vi "ComputeClassicalCrossTalk.vi"() -> ()   [LabVIEW 2015]
uses:
  <vilib>/Utility/file.llb/Write Delimited Spreadsheet (DBL).vi
panel:
  in  "stop":bool
  out "SLM  B":picture
  out "SLM A":picture
  out "Cross Talk":dbl[][](array[numeric])=[[1.04866638e-09, 2.36400149e-10, 3.28397032e-10, 3.4456285e-11, 1.42615789e-11, 6.36260558e-11, 1.65061454e-11, 1.20186092e-11, 3.22117194e-11, 4.34313557e-11, 1.69085523e-10, -3.68856204e-12, 5.28650778e-12, -1.44559289e-12, 7.52947704e-12, 3.04194213e-12, 9.77404269e-12, 3.04194213e-12, 7.52947704e-12, 7.98972867e-13, 3.04194213e-12], [1.0401547e-10, 2.07185158e-09, 5.01172714e-10, 4.89953078e-10, 3.66992547e-11, 9.77404269e-12, 4.34313557e-11, 5.46509886e-11, 9.77404269e-12, 6.81135912e-11, 1.51135382e-10, 6.81135912e-11, 9.05512679e-11, 1.87491134e-11, 1.0625844e-10, 2.77241841e-11, 1.20186092e-11, 4.1188386e-11, 5.28650778e-12, 1.20186092e-11, 3.04194213e-12], [3.57566809e-10, 2.61082406e-10, 4.32914238e-09, 1.01725206e-09, 9.49937462e-10, 1.2645314e-10, 1.65061454e-11, 7.93332275e-11, 8.38207628e-11, 5.68939583e-11, 5.01634567e-11, 9.77404269e-12, 4.1188386e-11, 1.42615789e-11, 2.77241841e-11, 1.65061454e-11, 9.77404269e-12, 1.20186092e-11, 7.52947704e-12, 1.65061454e-11, 9.77404269e-12], [5.28650778e-12, 7.52481022e-10, 3.50836304e-10, 9.81754322e-09, 2.47574095e-09, 1.2820246e-09, 2.880092e-10, 7.03581568e-11, 5.46509886e-11, 1.1523351e-10, 7.26011265e-11, 1.65061454e-11, 1.87491134e-11, 1.87491134e-11, 6.81135912e-11, 1.42615789e-11, 1.87491134e-11, 7.52947704e-12, 5.28650778e-12, 7.52947704e-12, 1.87491134e-11], [2.32366487e-11, 3.89438204e-11, 1.28651212e-09, 5.43805057e-10, 2.64532805e-08, 3.65150532e-09, 1.94619743e-09, 2.16205456e-10, 3.35129119e-10, 7.26011265e-11, 1.51135382e-10, 9.77404269e-12, 5.46509886e-11, 5.46509886e-11, 2.77241841e-11, 4.34313557e-11, 4.1188386e-11, 9.77404269e-12, 9.77404269e-12, 2.99687497e-11, 3.66992547e-11], [2.32366487e-11, 9.77404269e-12, 6.81135912e-11, 3.09503667e-09, 4.76490458e-10, 6.31465866e-08, 6.16683682e-09, 3.80632947e-09, 4.04688311e-10, 4.944406e-10, 2.70057476e-10, 7.70886618e-11, 4.1188386e-11, 4.34313557e-11, 2.32366487e-11, 7.93332275e-11, 1.65061454e-11, 7.98972867e-13, 5.28650778e-12, -1.44559289e-12, 7.52947704e-12], [2.77241841e-11, 9.77404269e-12, 8.60637325e-11, 6.81135912e-11, 4.02398204e-09, 5.52780155e-10, 1.38163287e-07, 1.08205347e-08, 5.81455462e-09, 9.25255206e-10, 3.19421961e-10, 3.66992547e-11, 3.04194213e-12, 9.72833689e-11, -1.44559289e-12, 4.1188386e-11, 3.4456285e-11, 7.52947704e-12, 3.22117194e-11, 1.87491134e-11, 5.28650778e-12], [-1.44559289e-12, 9.77404269e-12, 2.0993679e-11, 1.65061454e-11, 2.0993679e-11, 5.91777116e-09, 1.09578635e-09, 3.12278758e-07, 1.98609147e-08, 5.22442889e-09, 6.58690255e-11, 3.22117194e-11, 2.27425093e-10, 2.99687497e-11, 2.54812144e-11, 3.4456285e-11, 1.20186092e-11, 9.77404269e-12, 1.42615789e-11, 3.04194213e-12, 5.28650778e-12], [2.32366487e-11, 2.99687497e-11, 2.77241841e-11, 5.2406423e-11, 1.44403281e-10, 8.83082982e-11, 8.76070061e-09, 4.80707696e-09, 6.32152762e-07, 2.62266528e-08, 5.56100366e-09, 6.71703804e-10, 4.31613495e-10, 4.34313557e-11, 5.28650778e-12, 2.0993679e-11, 5.01634567e-11, 2.32366487e-11, 9.77404269e-12, 2.54812144e-11, 3.66992547e-11], [7.93332275e-11, 6.58690255e-11, 1.42615789e-11, 5.2406423e-11, 5.68939583e-11, 6.58690255e-11, 1.08503005e-10, 1.06881473e-08, 1.65898717e-09, 1.15755006e-06, 1.45834322e-08, 1.91702765e-09, 8.60637325e-11, 8.83082982e-11, 4.34313557e-11, 5.46509886e-11, 3.04194213e-12, 5.2406423e-11, 9.77404269e-12, 1.87491134e-11, 8.83082982e-11], [8.15761972e-11, 3.4456285e-11, 1.73573059e-10, 3.93468674e-10, 1.65061454e-11, 1.51135382e-10, 2.54812144e-11, 2.76789563e-10, 8.37476311e-09, 5.52285861e-09, 1.64707853e-06, 2.99917993e-08, 5.61755198e-10, 9.50388032e-11, 2.77241841e-11, 4.1188386e-11, 6.13814902e-11, 1.64597988e-10, 3.66992547e-11, 2.99687497e-11, 3.4456285e-11], [2.99687497e-11, 1.55622917e-10, -1.04206635e-11, 5.28650778e-12, 7.52947704e-12, 2.54812144e-11, 7.48456921e-11, 1.87035665e-10, 8.38207628e-11, 4.42786963e-09, 1.66796221e-09, 1.15531884e-06, 2.96282927e-08, 5.93169569e-10, 1.60110453e-10, 1.3542821e-10, 6.13814902e-11, 1.87491134e-11, 2.0993679e-11, 2.54812144e-11, 9.27958335e-11], [-1.44559289e-12, 1.20186092e-11, 3.66992547e-11, 7.52947704e-12, 3.22117194e-11, 2.32366487e-11, 6.13814902e-11, 1.42615789e-11, 2.81277113e-10, 3.37372102e-10, 2.21770047e-09, 2.88860535e-09, 6.35234073e-07, 1.90284553e-08, 6.87409407e-10, 4.15906365e-10, 4.34313557e-11, 2.0993679e-11, 6.81135912e-11, 3.04194213e-12, 4.1188386e-11], [9.77404269e-12, 5.28650778e-12, 2.99687497e-11, -1.44559289e-12, 3.4456285e-11, 2.54812144e-11, 9.95279345e-11, 3.4456285e-11, 9.95279345e-11, 1.87491134e-11, 4.944406e-10, 5.52780155e-10, 2.31642927e-09, 3.18151081e-07, 1.2180295e-08, 8.48965509e-10, 1.60110453e-10, 3.66992547e-11, 9.77404269e-12, 3.04194213e-12, 3.04194213e-12], [2.32366487e-11, 4.1188386e-11, 3.04194213e-12, 1.65061454e-11, 1.39915746e-10, 4.1188386e-11, 5.28650778e-12, 1.65061454e-11, 5.68939583e-11, 3.22117194e-11, 5.14635279e-10, 3.4456285e-11, 1.78060594e-10, 8.55697568e-10, 1.50108889e-07, 8.77640804e-09, 6.76191325e-10, 2.34157194e-10, 6.13814902e-11, 2.99687497e-11, 1.20186092e-11], [-3.68856204e-12, -8.17609695e-12, 9.77404269e-12, 1.87491134e-11, 3.89438204e-11, 1.42615789e-11, 7.93332275e-11, 2.0993679e-11, 1.28697705e-10, 9.05512679e-11, 4.78733442e-10, 3.35129119e-10, 1.10745975e-10, 1.0401547e-10, 3.03714776e-10, 7.20456086e-08, 4.18553636e-09, 6.08876727e-10, 1.21965604e-10, -3.68856204e-12, 2.77241841e-11], [2.54812144e-11, 9.77404269e-12, 2.54812144e-11, 2.99687497e-11, 6.13814902e-11, 9.77404269e-12, 2.54812144e-11, -8.17609695e-12, -1.44559289e-12, 7.03581568e-11, 3.26154048e-10, 7.93332275e-11, 5.46509886e-11, 1.19721039e-10, 6.13814902e-11, 4.3834561e-10, 3.08040633e-08, 2.34110997e-09, 4.29370539e-10, 9.77404269e-12, -3.68856204e-12], [1.42615789e-11, -8.17609695e-12, 2.77241841e-11, 9.77404269e-12, -8.17609695e-12, 5.46509886e-11, 2.77241841e-11, 4.1188386e-11, 7.52947704e-12, 7.98972867e-13, 2.99687497e-11, 1.12990541e-10, 2.32366487e-11, 1.20186092e-11, 1.42615789e-11, 9.50388032e-11, 3.5307926e-10, 1.28556854e-08, 9.18524701e-10, 3.48591739e-10, 3.04194213e-12], [7.98972867e-13, 1.87491134e-11, 7.98972867e-13, 2.0993679e-11, 2.0993679e-11, -3.68856204e-12, 3.66992547e-11, 1.42615789e-11, 1.42615789e-11, 1.65061454e-11, 2.25182123e-10, 3.04194213e-12, 6.58690255e-11, 7.98972867e-13, 3.04194213e-12, 1.65061454e-11, 1.3542821e-10, 1.55622917e-10, 2.99182012e-09, 5.37072997e-10, 2.27425093e-10], [3.04194213e-12, 5.28650778e-12, 5.28650778e-12, 3.4456285e-11, -3.68856204e-12, -8.17609695e-12, -1.44559289e-12, 1.42615789e-11, 5.91385205e-11, 1.42160311e-10, 1.24208574e-10, 8.15761972e-11, 1.20186092e-11, 7.52947704e-12, 5.28650778e-12, 5.01634567e-11, 1.42615789e-11, 3.66992547e-11, 9.72833689e-11, 2.95816283e-09, 2.04987402e-10], [1.20186092e-11, 9.77404269e-12, 2.54812144e-11, 1.42615789e-11, 5.28650778e-12, 1.87491134e-11, 1.42615789e-11, 7.52947704e-12, 5.28650778e-12, 1.65061454e-11, 1.42160311e-10, 5.2406423e-11, 2.77241841e-11, 1.65061454e-11, 1.42615789e-11, 3.04194213e-12, 1.42615789e-11, 7.98972867e-13, 2.54812144e-11, 9.27958335e-11, 1.53557755e-09]]
  out "Measured Power":dbl=1.53557755e-09
  out "Measured OAM Progress":u8(slide)=100 scale=0.0..100.0
  out "Generated OAM Progress":u8(slide)=100 scale=0.0..100.0
  out "Current Measured OAM":i32=10
  out "Current Generated OAM":i32=10
  in  "Measured OAM":i32[](array[numeric])=[-10, -9, -8, -7, -6, -5, -4, -3, -2, -1, 0, 1, 2, 3, 4, 5, 6, 7, 8, 9, 10]
  in  "Generated OAM":i32[](array[numeric])=[-10, -9, -8, -7, -6, -5, -4, -3, -2, -1, 0, 1, 2, 3, 4, 5, 6, 7, 8, 9, 10]
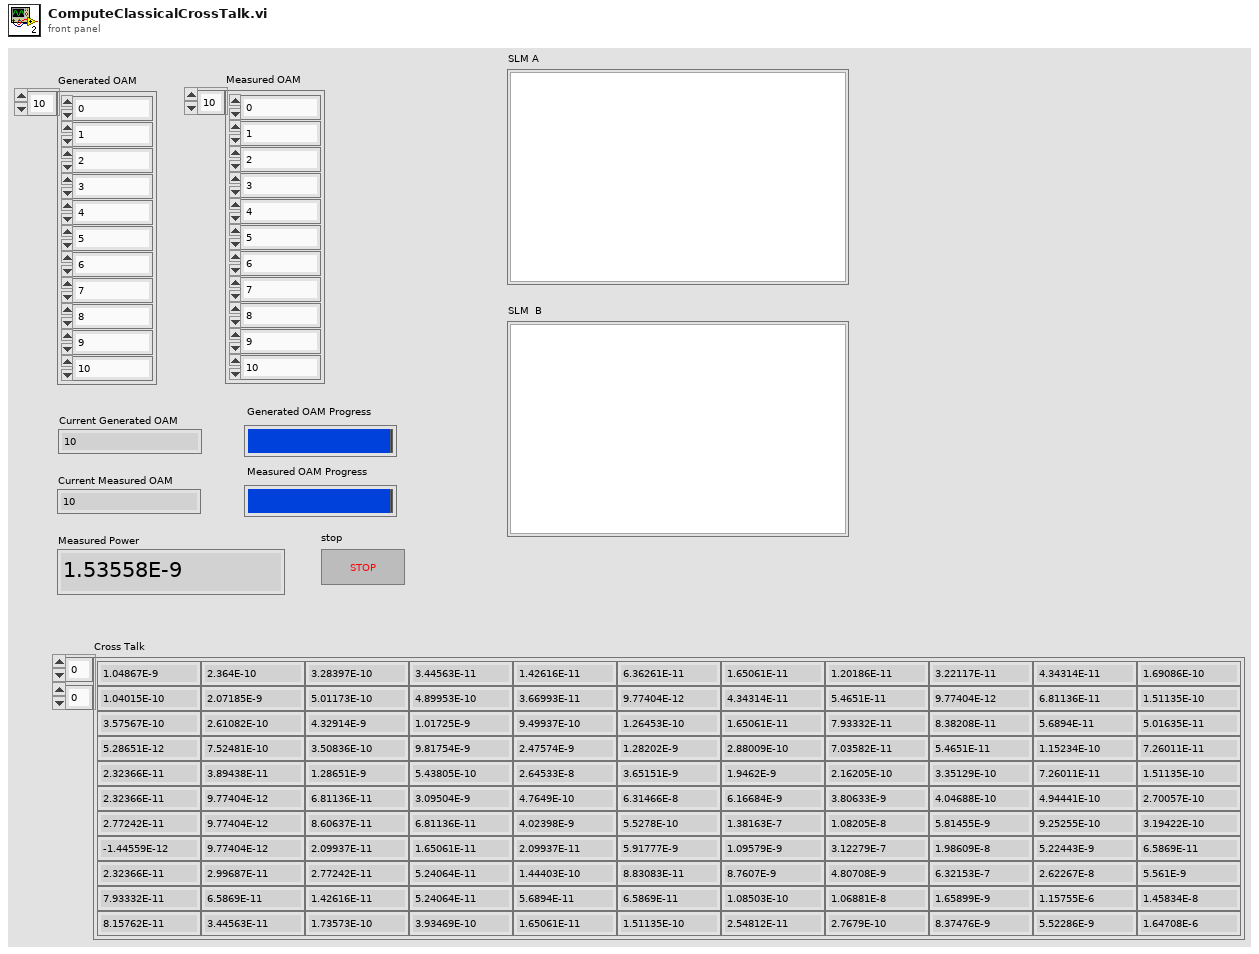
[diagram p1: front panel]
types:
  T1 = cluster{"type":enum16{"Azimuth Mode", "LG mode", "HG mode"}, "Numeric":i32, i32, dbl, dbl}
  T2 = cluster{"type":enum16{"Azimuth Mode", "LG mode", "HG mode"}, "Numeric":i32, i32, dbl, dbl}[]
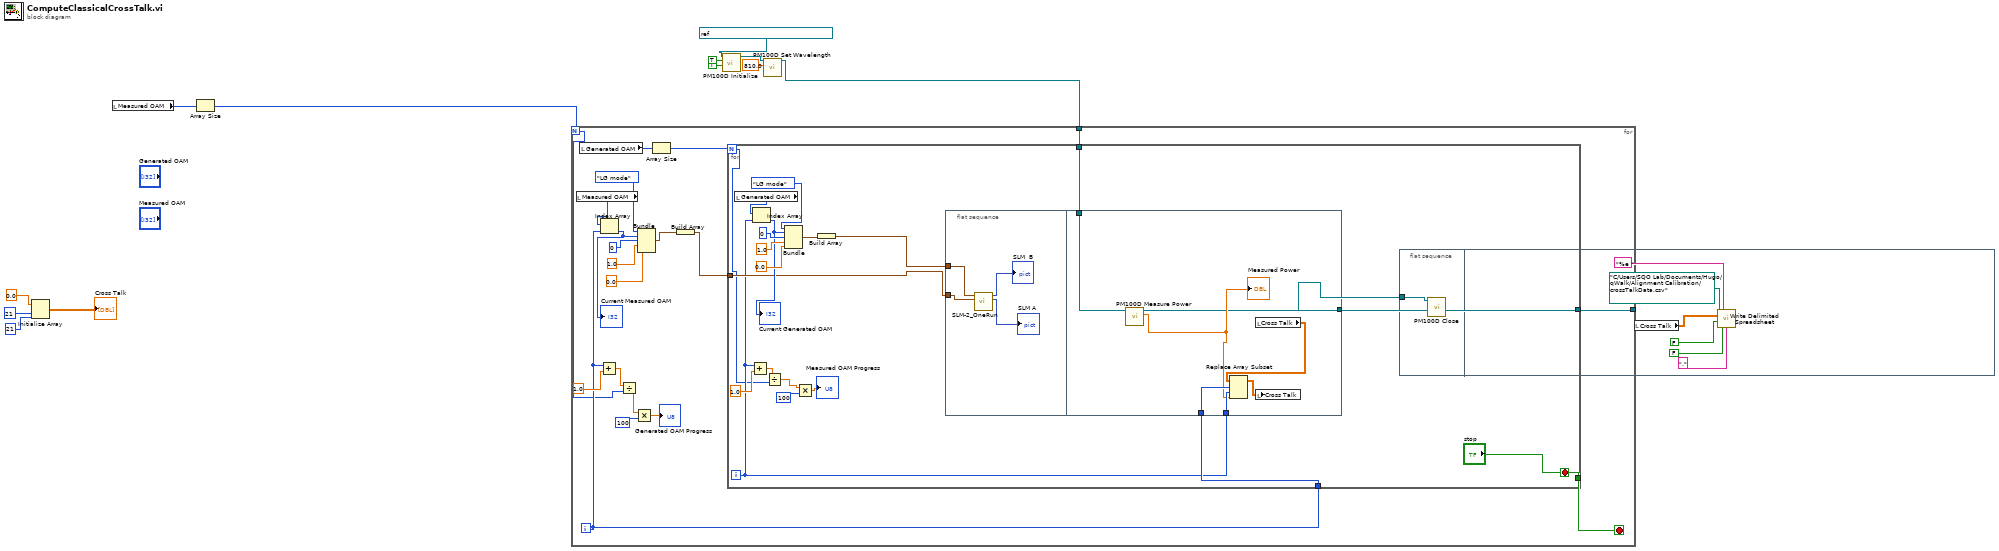
[diagram p0: block diagram]
diagram:
  n1 = Initialize Array(0.0 ("element"), 21 ("dimension size"), 21 ("dimension size")) -> (→"Cross Talk":dbl[][])
  n2 = local read "Measured OAM"() -> (w13:i32[])
  n3 = Array Size(array=w13) -> (size(s)=w12:i32)
  n4 = call <instrlib>:"PM100D Initialize.vi"("Reset Device (Reset Device)"=TRUE, "ID Query (Do Query)"=TRUE, "resource name"=refnum<visa-resource-name> "USB0::0x1313::0x8078::P0003776::INSTR") -> ("instrument handle out"=w10:refnum<visa-resource-name>)  [unwired: 7 in, 1 out]
  n5 = call <instrlib>:"PM100D Set Wavelength.vi"("Wavelength (0.0)"=810.0, "instrument handle"=w10) -> ("instrument handle out"=w6:refnum<visa-resource-name>)  [unwired: 8 in, 1 out]
  n6 = for {
    N: w12 -> [w16]
    tunnel: w6 -> [w21]
    tunnel: [w20] -> w1
    i -> [w18]
    stop <- w14 stop-if-true
    n7 = local read "Measured OAM"() -> (w31:i32[])
    n8 = local read "Generated OAM"() -> (w33:i32[])
    n9 = Add(x=w18, y=1.0) -> (x+y=w17:dbl)
    n10 = Index Array(array=w31, index=w18) -> (element=w26:i32)
    "Current Measured OAM" <- w26
    n11 = Divide(x=w17, y=w16) -> (x/y=w15:dbl)
    n12 = Multiply(x=w15, y=100) -> (x*y=→"Generated OAM Progress":dbl)
    n13 = Bundle("type"=enum16{"Azimuth Mode", "LG mode", "HG mode"}."LG mode", "Numeric"=w26, 0, 1.0, 0.0) -> (w23:T1)  [unwired: 1 in]
    n14 = Array Size(array=w33) -> (size(s)=w32:i32)
    n15 = Build Array(w23) -> (w22:T2)
    n16 = for {
      N: w32 -> [w36]
      tunnel: w22 -> [w42]
      tunnel: w18 -> [w44]
      tunnel: w21 -> [w40]
      tunnel: [w39] -> w20
      tunnel: ["stop"] -> w14
      i -> [w38]
      stop <- "stop" stop-if-true
      n17 = local read "Generated OAM"() -> (w53:i32[])
      n18 = Add(x=w38, y=1.0) -> (x+y=w35:dbl)
      n19 = Index Array(array=w53, index=w38) -> (element=w46:i32)
      "Current Generated OAM" <- w46
      n20 = Divide(x=w35, y=w36) -> (x/y=w37:dbl)
      n21 = Bundle("type"=enum16{"Azimuth Mode", "LG mode", "HG mode"}."LG mode", "Numeric"=w46, 0, 1.0, 0.0) -> (w45:T1)  [unwired: 1 in]
      n22 = Multiply(x=w37, y=100) -> (x*y=→"Measured OAM Progress":dbl)
      n23 = Build Array(w45) -> (w43:T2)
      n24 = flat-sequence {
        tunnel: w43 -> [w57]
        tunnel: w42 -> [w56]
        tunnel: w44 -> [w62]
        tunnel: w38 -> [w61]
        tunnel: w40 -> [w59]
        tunnel: [w58] -> w39
        frame #0 {
          n25 = call "SLM-2_OneRun.vi"("Modes B - SLM 2"=w56, "Modes - UV"=w57) -> ("SLM"=→"SLM A":picture, "SLM  B"=→"SLM  B":picture)  [unwired: 8 in]
        }
        frame #1 {
          n26 = call <instrlib>:"PM100D Measure Power.vi"("instrument handle"=w59) -> ("Power"=w60:dbl, "instrument handle out"=w58:refnum<visa-resource-name>)  [unwired: 8 in, 1 out]
          "Measured Power" <- w60
          n27 = local read "Cross Talk"() -> (w64:dbl[][])
          n28 = Replace Array Subset(array=w64, new element=w60, index (row)=w62, index (col)=w61) -> (w63:dbl[][])
          n29 = local write "Cross Talk"(w63) -> ()
        }
      }
    }
  }
  n30 = flat-sequence {
    tunnel: w1 -> [w65]
    frame #0 {
      n31 = call <instrlib>:"PM100D Close.vi"("instrument handle"=w65) -> ()  [unwired: 10 in, 1 out]
    }
    frame #1 {
      n32 = local read "Cross Talk"() -> (w66:dbl[][])
      n33 = call-poly <vilib>:"Write Delimited Spreadsheet.vi"("file path (dialog if empty)"=path "C:/Users/SQO Lab/Documents/Hugo/qWalk/Alignment Calibration/crossTalkData.csv", "format (%.3f)"="%e ", "2D data"=w66, "append to file? (F)"=FALSE, "transpose? (F)"=FALSE, "delimiter (\\t)"=",") -> ()  [unwired: 8 in, 2 out]
    }
  }
